vi "动态优化_新.vi"(4 "S_CCw":dbl[](array[numeric]), 5 "S_Cw":dbl[](array[numeric]), 6 "P_CCw":dbl[](array[numeric]), 7 "SENSOR":T1, 8 "P_Cw":dbl[](array[numeric]), 9 "T2_AV(%)":dbl, 10 "T1_AV(%)":dbl) -> (3 "OK？":bool)   [LabVIEW 2020]
uses:
  Global_Variable/Global.vi
panel:
  out "Temp1":dbl
  out "Temp":dbl
  out "S(%)":dbl
  out "P(%)":dbl
  out "PROC_1":i32
  out "T2ROC1+T2ROC2+T2ROC3":i32
  out "T1ROC1+T1ROC2+T1ROC3":i32
  out "T2ROC_3":i32
  out "T1ROC_3":i32
  out "T2ROC_2":i32
  out "T1ROC_2":i32
  out "PROC":i32
  out "error out":errorcluster caption="错误输出"
  in  "error in (no error)":errorcluster caption="错误输入（无错误）"
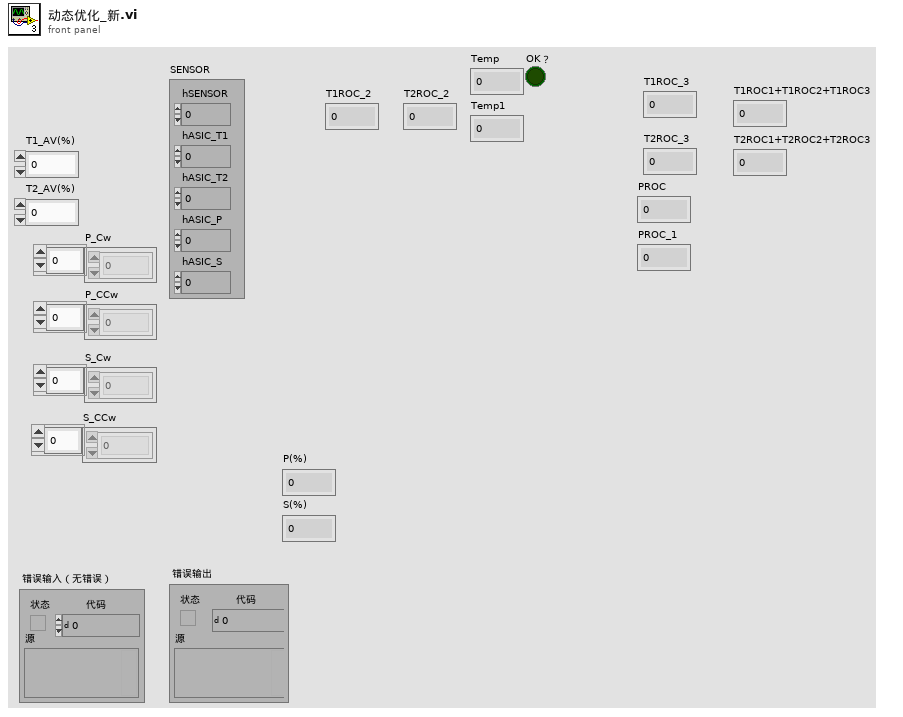
[diagram p1: front panel]
types:
  T1 = cluster{"hSENSOR":i32, "hASIC_T1":i32, "hASIC_T2":i32, "hASIC_P":i32, "hASIC_S":i32}
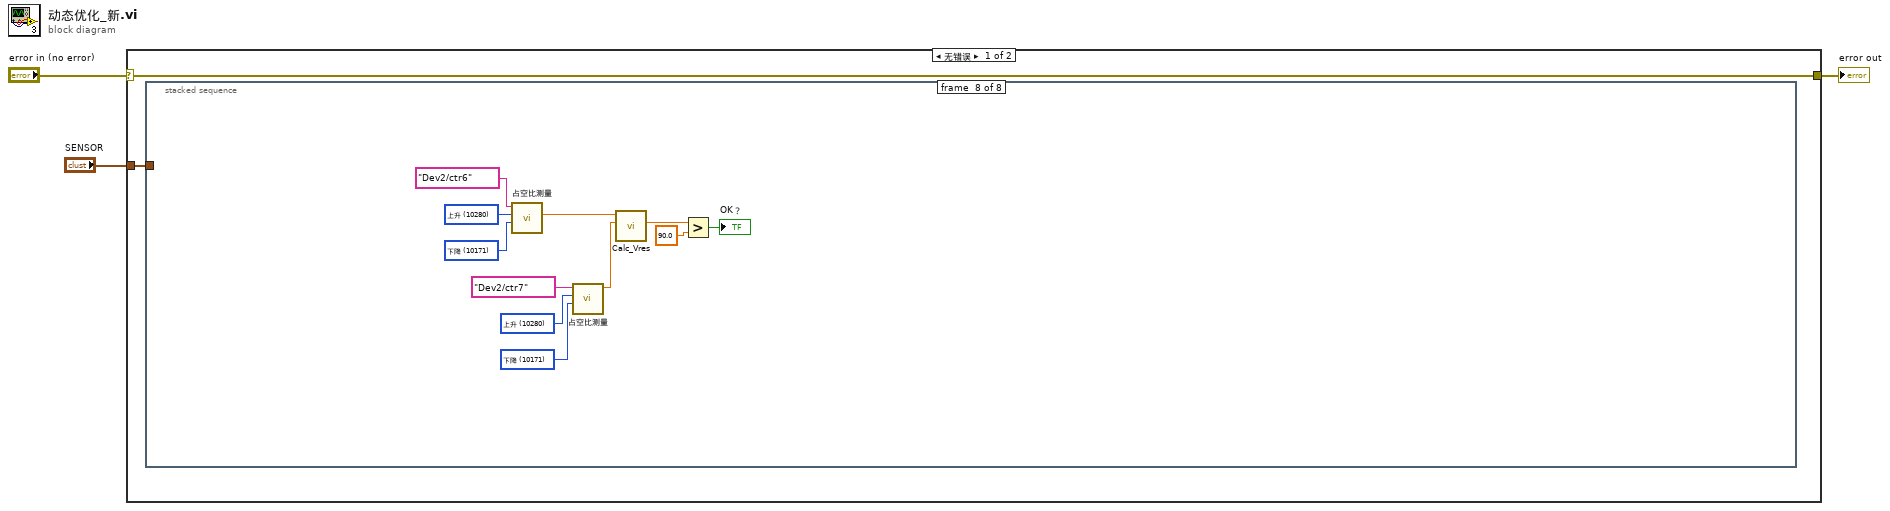
[diagram p0: block diagram]
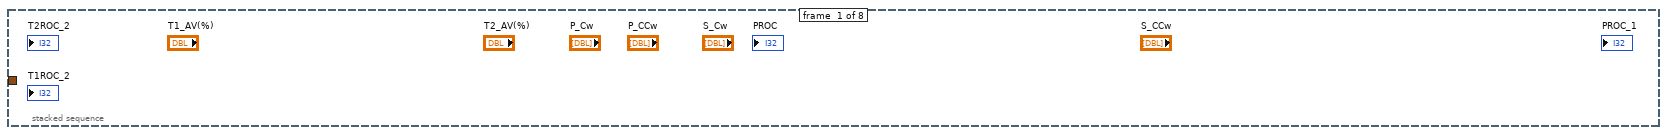
[diagram p2: hidden frame]
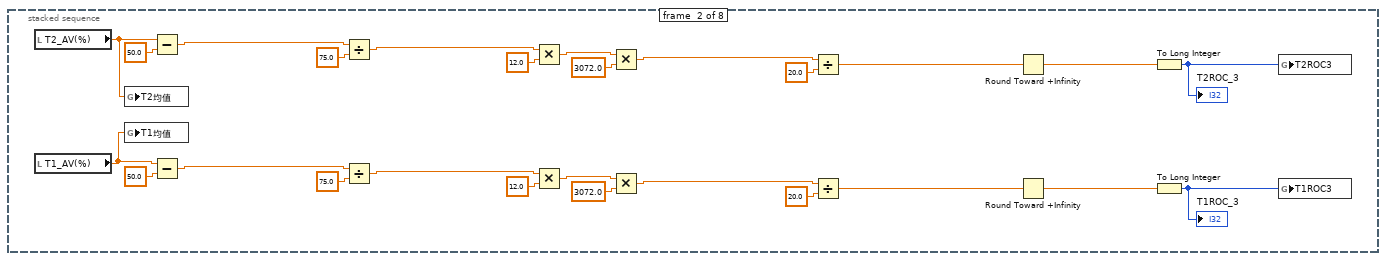
[diagram p3: hidden frame]
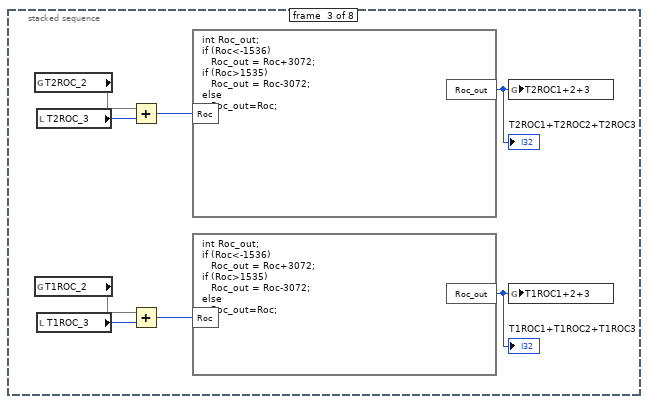
[diagram p4: hidden frame]
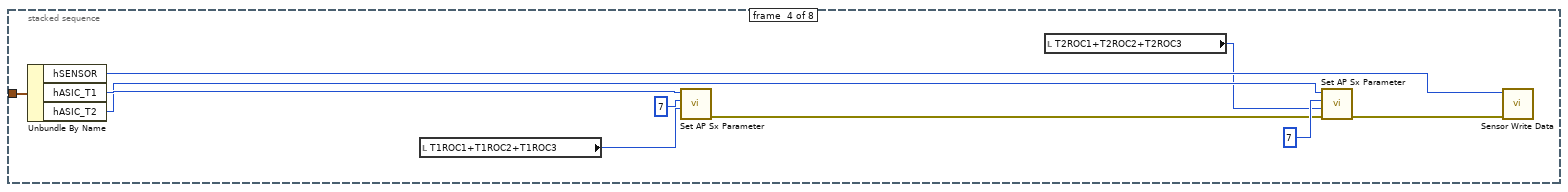
[diagram p5: hidden frame]
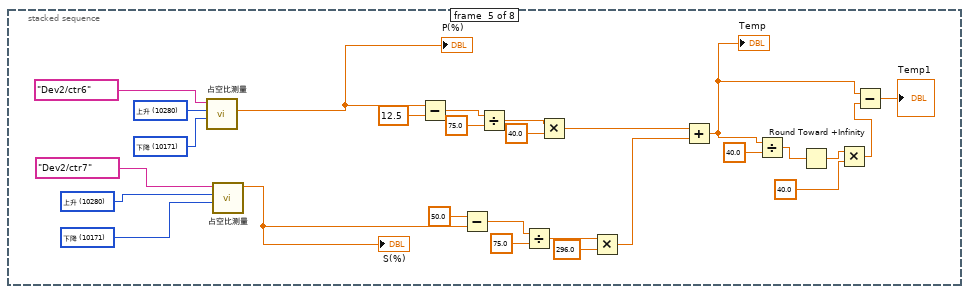
[diagram p6: hidden frame]
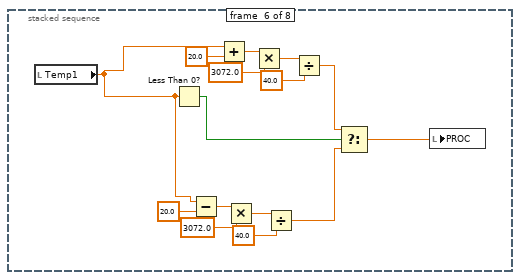
[diagram p7: hidden frame]
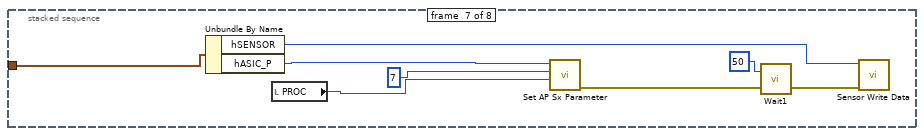
[diagram p8: hidden frame]
diagram:
  n1 = case shown="无错误" "error in (no error)" {
    selector: "error in (no error)" -> [w4 w111]
    tunnel: [w4 w111] -> w2
    tunnel: "SENSOR" -> [w5 _]
    frame No Error {
      n2 = stacked-sequence {
        tunnel: w5 -> [_ _ _ w49 _ _ w92 _]
        frame #0 {
        }
        frame #1 {
          n3 = local read "T2_AV(%)"() -> (w6:dbl)
          n4 = local read "T1_AV(%)"() -> (w7:dbl)
          n5 = global write "Global.vi" "T2均值"(w6) -> ()
          n6 = global write "Global.vi" "T1均值"(w7) -> ()
          n7 = Subtract(x=w6, y=50.0) -> (x-y=w19:dbl)
          n8 = Subtract(x=w7, y=50.0) -> (x-y=w30:dbl)
          n9 = Divide(x=w19, y=75.0) -> (x/y=w21:dbl)
          n10 = Divide(x=w30, y=75.0) -> (x/y=w28:dbl)
          n11 = Multiply(x=w21, y=12.0) -> (x*y=w16:dbl)
          n12 = Multiply(x=w28, y=12.0) -> (x*y=w15:dbl)
          n13 = Multiply(x=w16, y=3072.0) -> (x*y=w14:dbl)
          n14 = Multiply(x=w15, y=3072.0) -> (x*y=w13:dbl)
          n15 = Divide(x=w14, y=20.0) -> (x/y=w12:dbl)
          n16 = Divide(x=w13, y=20.0) -> (x/y=w17:dbl)
          n17 = Round Toward +Infinity(x=w12) -> (ceil(x): smallest int >= x=w11:dbl)
          n18 = Round Toward +Infinity(x=w17) -> (ceil(x): smallest int >= x=w10:dbl)
          n19 = To Long Integer(number=w11) -> (32bit integer=w8:i32)
          "T2ROC_3" <- w8
          n20 = To Long Integer(number=w10) -> (32bit integer=w9:i32)
          "T1ROC_3" <- w9
          n21 = global write "Global.vi" "T2ROC3"(w8) -> ()
          n22 = global write "Global.vi" "T1ROC3"(w9) -> ()
        }
        frame #2 {
          n23 = global read "Global.vi" "T2ROC_2"() -> (w32)
          n24 = global read "Global.vi" "T1ROC_2"() -> (w33)
          n25 = local read "T2ROC_3"() -> (w36:i32)
          n26 = local read "T1ROC_3"() -> (w39:i32)
          n27 = Add(x=w32, y=w36) -> (x+y=w37:i32)
          n28 = Add(x=w33, y=w39) -> (x+y=w38:i32)
          n29 = formula code="int Roc_out;\nif (Roc<-1536)\n   Roc_out = Roc+3072;\nif (Roc>1535)\n   Roc_out = Roc-3072;\nelse\n   Roc_out=Roc;"("Roc"=w37) -> ("Roc_out"=w34:i32)
          "T2ROC1+T2ROC2+T2ROC3" <- w34
          n30 = formula code="int Roc_out;\nif (Roc<-1536)\n   Roc_out = Roc+3072;\nif (Roc>1535)\n   Roc_out = Roc-3072;\nelse\n   Roc_out=Roc;"("Roc"=w38) -> ("Roc_out"=w35:i32)
          "T1ROC1+T1ROC2+T1ROC3" <- w35
          n31 = global write "Global.vi" "T2ROC1+2+3"(w34) -> ()
          n32 = global write "Global.vi" "T1ROC1+2+3"(w35) -> ()
        }
        frame #3 {
          n33 = Unbundle By Name(w49) -> ("hSENSOR"=w46:i32, "hASIC_T1"=w48:i32, "hASIC_T2"=w47:i32)
          n34 = local read "T1ROC1+T1ROC2+T1ROC3"() -> (w41:i32)
          n35 = call "Set AP Sx Parameter.vi"("para2"=w41, "asicBitsName"=7, "asicHandle"=w48) -> ("error out"=w43:errorcluster)  [unwired: 7 in, 1 out]
          n36 = local read "T2ROC1+T2ROC2+T2ROC3"() -> (w40:i32)
          n37 = call "Set AP Sx Parameter.vi"("error in (no error)"=w43, "para2"=w40, "asicBitsName"=7, "asicHandle"=w47) -> ("error out"=w42:errorcluster)  [unwired: 6 in, 1 out]
          n38 = call "Sensor Write Data.vi"("error in (no error)"=w42, "sensorHandle"=w46) -> ()  [unwired: 8 in, 2 out]
        }
        frame #4 {
          w71 = 10171 items=["上升"=10280, "下降"=10171] ("starting edge2")
          w72 = 10280 items=["上升"=10280, "下降"=10171] ("starting edge1")
          w73 = 10171 items=["上升"=10280, "下降"=10171] ("starting edge2")
          w74 = 10280 items=["上升"=10280, "下降"=10171] ("starting edge1")
          n39 = call "占空比测量.vi"("计数器"=tag "Dev2/ctr6", "starting edge1"=w74, "starting edge2"=w73) -> ("占空比2(%)"=w70:dbl)  [unwired: 4 in, 3 out]
          "P(%)" <- w70
          n40 = call "占空比测量.vi"("计数器"=tag "Dev2/ctr7", "starting edge1"=w72, "starting edge2"=w71) -> ("占空比(%)"=w64:dbl)  [unwired: 4 in, 3 out]
          "S(%)" <- w64
          n41 = Subtract(x=w70, y=12.5) -> (x-y=w68:dbl)
          n42 = Subtract(x=50.0, y=w64) -> (x-y=w61:dbl)
          n43 = Divide(x=w68, y=75.0) -> (x/y=w66:dbl)
          n44 = Divide(x=w61, y=75.0) -> (x/y=w59:dbl)
          n45 = Multiply(x=w66, y=40.0) -> (x*y=w62:dbl)
          n46 = Multiply(x=w59, y=296.0) -> (x*y=w57:dbl)
          n47 = Add(x=w62, y=w57) -> (x+y=w56:dbl)
          "Temp" <- w56
          n48 = Divide(x=w56, y=40.0) -> (x/y=w54:dbl)
          n49 = Round Toward +Infinity(x=w54) -> (ceil(x): smallest int >= x=w53:dbl)
          n50 = Multiply(x=w53, y=40.0) -> (x*y=w51:dbl)
          n51 = Subtract(x=w56, y=w51) -> (x-y=→"Temp1":dbl)
        }
        frame #5 {
          n52 = local read "Temp1"() -> (w79:dbl)
          n53 = Less Than 0?(x=w79) -> (x < 0?=w91:bool)
          n54 = Subtract(x=w79, y=20.0) -> (x-y=w81:dbl)
          n55 = Add(x=w79, y=20.0) -> (x+y=w89:dbl)
          n56 = Multiply(x=w81, y=3072.0) -> (x*y=w83:dbl)
          n57 = Multiply(x=w89, y=3072.0) -> (x*y=w87:dbl)
          n58 = Divide(x=w83, y=40.0) -> (x/y=w78:dbl)
          n59 = Divide(x=w87, y=40.0) -> (x/y=w85:dbl)
          n60 = Select(t=w85, s=w91, f=w78) -> (s? t:f=w77:dbl)
          n61 = local write "PROC"(w77) -> ()
        }
        frame #6 {
          n62 = Unbundle By Name(w92) -> ("hSENSOR"=w98:i32, "hASIC_P"=w99:i32)
          n63 = local read "PROC"() -> (w95:i32)
          n64 = call "Set AP Sx Parameter.vi"("para2"=w95, "asicBitsName"=7, "asicHandle"=w99) -> ("error out"=w97:errorcluster)  [unwired: 7 in, 1 out]
          n65 = call "Wait1.vi"("error in (no error)"=w97, "Wait（150ms）"=u32 50) -> ("error out"=w96:errorcluster)  [unwired: 1 in]
          n66 = call "Sensor Write Data.vi"("error in (no error)"=w96, "sensorHandle"=w98) -> ()  [unwired: 8 in, 2 out]
        }
        frame #7 {
          w108 = 10171 items=["上升"=10280, "下降"=10171] ("starting edge2")
          w109 = 10280 items=["上升"=10280, "下降"=10171] ("starting edge1")
          w105 = 10171 items=["上升"=10280, "下降"=10171] ("starting edge2")
          w106 = 10280 items=["上升"=10280, "下降"=10171] ("starting edge1")
          n67 = call "占空比测量.vi"("计数器"=tag "Dev2/ctr6", "starting edge1"=w106, "starting edge2"=w105) -> ("占空比2(%)"=w104:dbl)  [unwired: 4 in, 3 out]
          n68 = call "占空比测量.vi"("计数器"=tag "Dev2/ctr7", "starting edge1"=w109, "starting edge2"=w108) -> ("占空比(%)"=w103:dbl)  [unwired: 4 in, 3 out]
          n69 = call "Calc_Vres.vi"("S_Data in"=w103, "P_Data in"=w104) -> ("Vres"=w102:dbl)  [unwired: 7 in, 2 out]
          n70 = Greater?(x=w102, y=90.0) -> (0:→"OK？":bool)
        }
      }
    }
    frame Error {
    }
  }
  "error out" <- w2
